vi "Parse Auto Data.vi"(11 "path":path) -> (1 "Zero Velocity?":bool[](array[boolean]), 2 "Velocities":T3[](array[typedef]), 3 "Positions":cluster{"x":dbl, "y":dbl, "th":dbl}[](array[cluster]), 5 "Commands out":cluster{"Time (s)":dbl, T1, bool}[](array[cluster]), 7 "Overall":cluster{"Time (s)":dbl, "Distance (ft)":dbl})   [LabVIEW 2025]
uses:
  swerve-template/Type Definitions/Data/Robot Velocities.ctl
  bordeaux/Bordeaux/Types/Single Cmd Info.ctl
  <vilib>/picture/picture.llb/imagedata.ctl
  <vilib>/Analysis/coordinate.llb/2D Cartesian Coordinate Rotation (Scalar).vi
  <vilib>/Analysis/NI_AALPro.lvlib
panel:
  in  "Is Blue Alliance":bool=TRUE
  out "XY Graph":cluster{dbl[], dbl[]}[](graph)
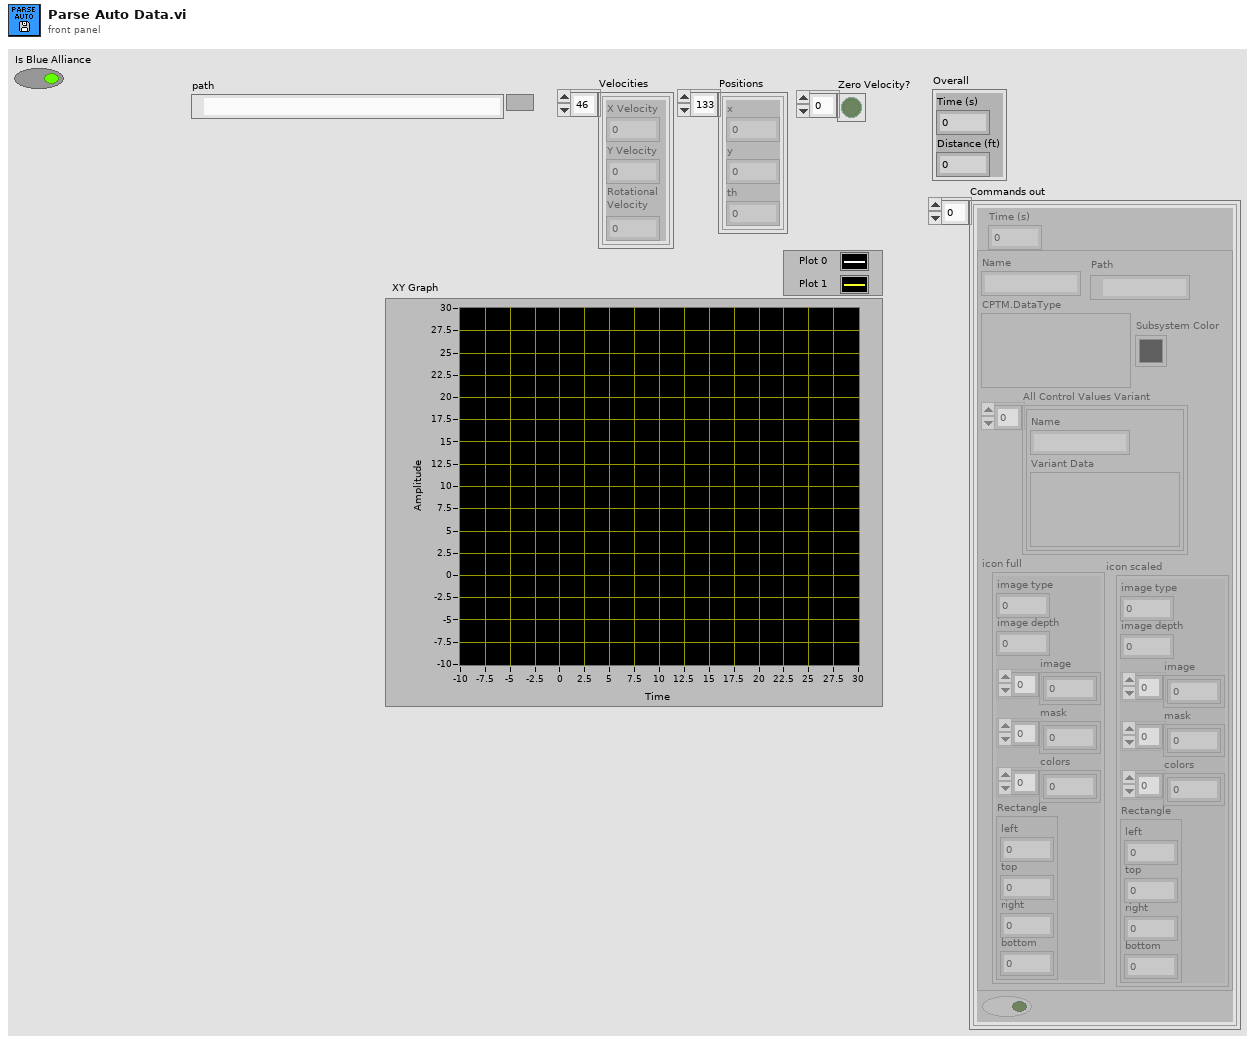
[diagram p1: front panel]
types:
  T1 = typedef "Single Cmd Info.ctl" = cluster{"Name":string, "CPTM.DataType":variant, "All Control Values Variant":cluster{"Name":string, "Variant Data":variant}[], "icon full":T2, "icon scaled":T2, "Path":path, "Subsystem Color":u32}
  T2 = typedef "imagedata.ctl" = cluster{"image type":i32, "image depth":i32, "image":u8[], "mask":u8[], "colors":u32[], "Rectangle":cluster{"left":i16, "top":i16, "right":i16, "bottom":i16}}
  T3 = typedef "Robot Velocities.ctl" = cluster{"X Velocity":dbl, "Y Velocity":dbl, "Rotational \nVelocity":dbl}
  T4 = typedef "Trajectory Data.ctl" = cluster{"Segment Name":string, "Type":T5, "Traj Pos Points":cluster{"x":dbl, "y":dbl, "th":dbl}[], "Traj Vel Points":cluster{"V":dbl, "Omega":dbl, "V vector":cluster{"y":dbl, "x":dbl}}[], "Accel Index":i32, "Decel Index":i32}[]
  T5 = typedef "Segment Type.ctl" = enum16{"Accel Straight", "Const Straight", "Blend", "Circle", "Bezier"}
  T6 = typedef "WPI_DriverStationAllianceInfo.ctl" = enum16{"Red", "Blue", "Invalid"}
  T7 = cluster{"V":dbl, "Omega":dbl, "V vector":cluster{"y":dbl, "x":dbl}}[]
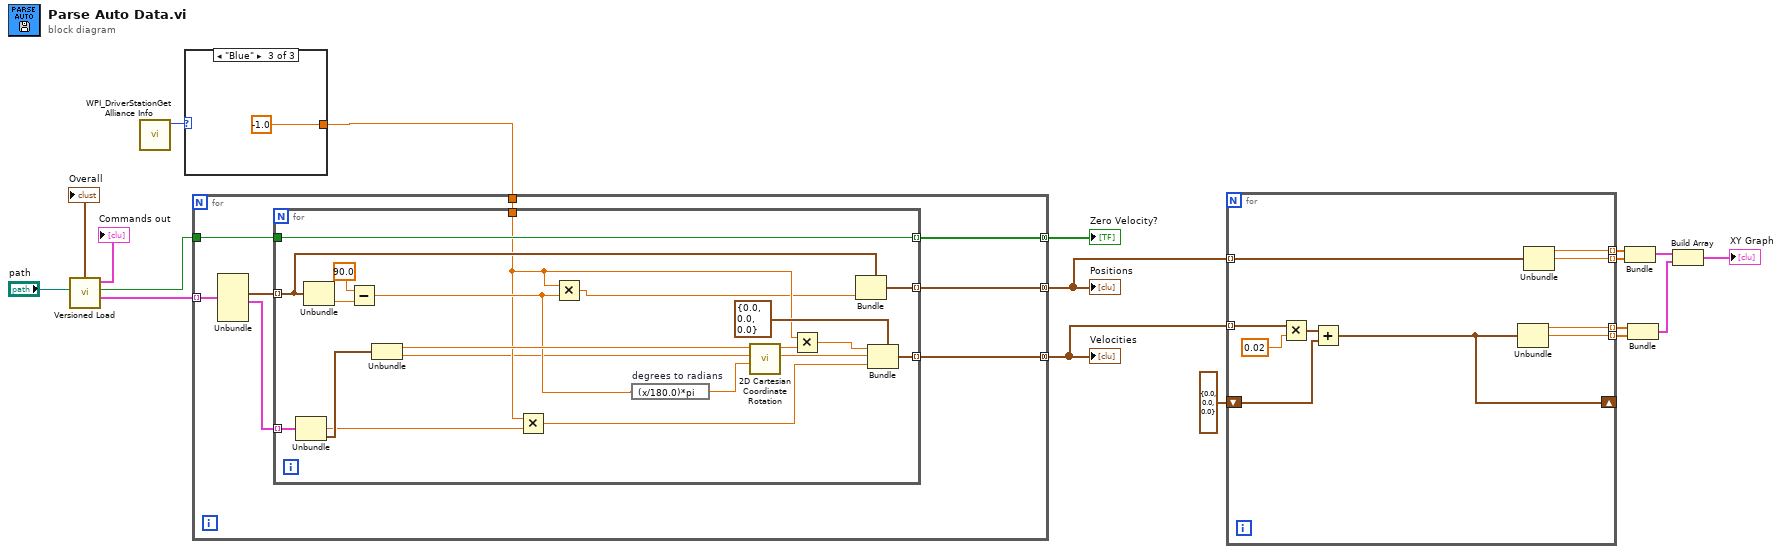
[diagram p0: block diagram]
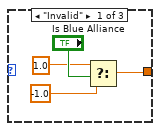
[diagram p2: hidden frame]
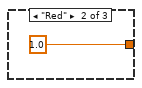
[diagram p3: hidden frame]
diagram:
  n1 = call "Versioned Load.vi"("path"="path") -> ("Trajectory Data"=w18:T4, "Zero V"=w17:bool, "Commands out"=→"Commands out":cluster{"Time (s)":dbl, T1, bool}[], "Overall"=→"Overall":cluster{"Time (s)":dbl, "Distance (ft)":dbl})  [unwired: 3 in, 4 out]
  n2 = call <vilib>:"WPI_DriverStationGet Alliance Info.vi"() -> ("Alliance"=w2:T6)  [unwired: 6 in, 5 out]
  n3 = case shown="\"Blue\"" w2 {
    tunnel: [w19 1.0 -1.0] -> w1
    frame "Invalid" {
      n4 = Select(t=1.0, s="Is Blue Alliance", f=-1.0) -> (s? t:f=w19:dbl)
    }
    frame "Red" {
    }
    frame "Blue" {
    }
  }
  n5 = for {
    tunnel: w18 -> [w32] mode=indexing
    tunnel: [w29] -> w14 mode=concatenating
    tunnel: w1 -> [w28]
    tunnel: [w25] -> w13 mode=concatenating
    tunnel: w17 -> [w27]
    tunnel: [w26] -> w16 mode=concatenating
    n6 = Unbundle(w32) -> ("Traj Pos Points"=w31:cluster{"x":dbl, "y":dbl, "th":dbl}[], "Traj Vel Points"=w30:T7)  [unwired: 4 out]
    n7 = for {
      tunnel: w31 -> [w50] mode=indexing
      tunnel: w30 -> [w48] mode=indexing
      tunnel: [w49] -> w29 mode=indexing
      tunnel: w28 -> [w36]
      tunnel: [w41] -> w25 mode=indexing
      tunnel: w27 -> [w38]
      tunnel: [w38] -> w26 mode=indexing
      n8 = Unbundle(w48) -> ("Omega"=w34:dbl, "V vector"=w47:cluster{"y":dbl, "x":dbl})  [unwired: 1 out]
      n9 = Unbundle(w50) -> ("th"=w52:dbl)  [unwired: 2 out]
      n10 = Subtract(x=90.0, y=w52) -> (x-y=w37:dbl)
      n11 = Unbundle(w47) -> ("y"=w45:dbl, "x"=w33:dbl)
      n12 = Multiply(x=w36, y=w34) -> (x*y=w43:dbl)
      n13 = Multiply(x=w36, y=w37) -> (x*y=w35:dbl)
      n14 = expression code="(x/180.0)*pi" "degrees to radians"(w37) -> (w46:dbl)
      n15 = call-poly <vilib>:"2D Cartesian Coordinate Rotation.vi"("theta"=w46, "y"=w33, "x"=w45) -> ("y out"=w44:dbl, "x out"=w40:dbl)  [unwired: 6 in, 1 out]
      n16 = Multiply(x=w36, y=w40) -> (x*y=w39:dbl)
      n17 = Bundle(cluster=w50, "th"=w35) -> (w49:cluster{"x":dbl, "y":dbl, "th":dbl})  [unwired: 2 in]
      n18 = Bundle(cluster=T3 {"X Velocity"=0.0, "Y Velocity"=0.0, "Rotational \nVelocity"=0.0} ("Robot Velocities"), "X Velocity"=w39, "Y Velocity"=w44, "Rotational \nVelocity"=w43) -> (w41:T3)
    }
  }
  "Positions" <- w14
  "Velocities" <- w13
  "Zero Velocity?" <- w16
  n19 = for {
    tunnel: w14 -> [w62] mode=indexing
    tunnel: w13 -> [w59] mode=indexing
    tunnel: [w61] -> w12 mode=indexing
    tunnel: [w60] -> w11 mode=indexing
    shift-right: [w55] -> _
    shift-left: T3 {"X Velocity"=0.0, "Y Velocity"=0.0, "Rotational \nVelocity"=0.0} ("Robot Velocities") -> [w56]
    tunnel: [w54] -> w9 mode=indexing
    tunnel: [w53] -> w8 mode=indexing
    n20 = Multiply(x=w59, y=0.02) -> (x*y=w57:T3)
    n21 = Add(x=w57, y=w56) -> (x+y=w55:T3)
    n22 = Unbundle(w55) -> ("X Velocity"=w54:dbl, "Y Velocity"=w53:dbl)  [unwired: 1 out]
    n23 = Unbundle(w62) -> ("x"=w61:dbl, "y"=w60:dbl)  [unwired: 1 out]
  }
  n24 = Bundle(w12, w11) -> (w7:cluster{dbl[], dbl[]})  [unwired: 1 in]
  n25 = Bundle(w9, w8) -> (w6:cluster{dbl[], dbl[]})  [unwired: 1 in]
  n26 = Build Array(w7, w6) -> (→"XY Graph":cluster{dbl[], dbl[]}[])
